vi "Write fileContentsString.vi"(10 "fileContentsString":string, 11 "IDLFile in":refnum<class "IDLFile.lvclass">) -> (3 "IDLFile out":refnum<class "IDLFile.lvclass">)   [LabVIEW 2012, in "IDLFile.lvclass"]
uses:
  IDLFile.lvclass
  IDLFile.lvclass/IDLFile.ctl
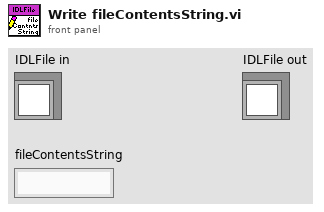
[diagram p1: front panel]
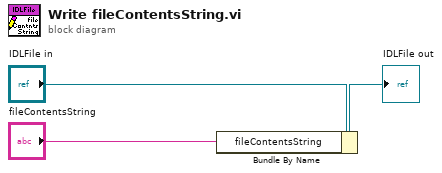
[diagram p0: block diagram]
diagram:
  n1 = Bundle By Name(cluster="IDLFile in", "fileContentsString"="fileContentsString") -> (→"IDLFile out":refnum<class "IDLFile.lvclass">)
